vi "ProyectoFinal.vi"() -> ()   [LabVIEW 2020]
uses:
  <vilib>/Instr/_visa.llb/VISA Configure Serial Port (Instr).vi
panel:
  in  "Temperatura Base":string
  out "Unidades de calor":dbl
  in  "Escribir":bool
  in  "Leer":bool
  out "Concentracion de CO":dbl
  out "Temperatura actual":dbl
  out "Humedad actual":dbl
  in  "Temperatura deseada":string
  in  "humedad deseada":string
  in  "VISA resource name":refnum<visa-resource-name>
  in  "stop":bool
  # "INSTITUTO POLITECNICO NACIONAL \nUNIDAD PROFECIONAL INTERDICIPLINARIA DE INGIENERIA CAMPUS ZACATECAS \nPROYECTO: INVERNADERO \nINSTRUMENTACION VIRTUAL"
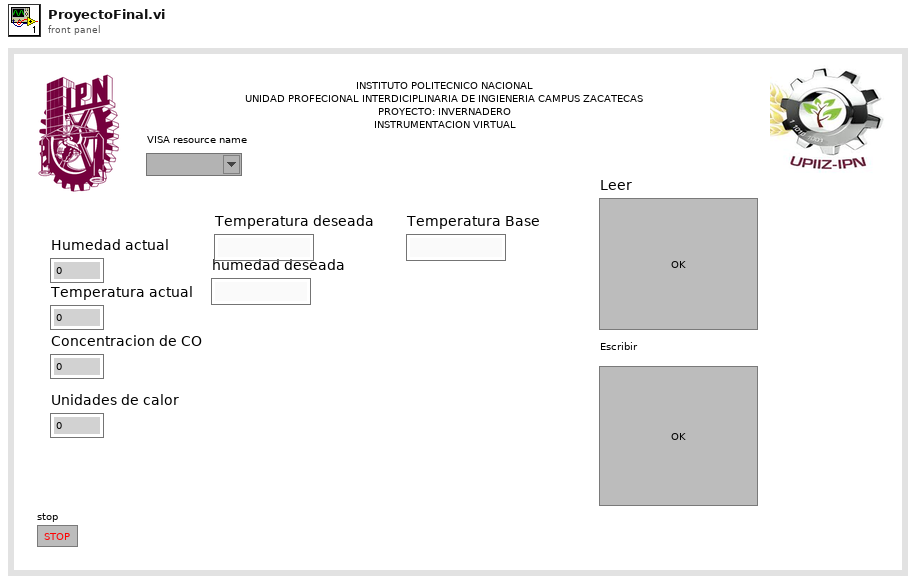
[diagram p1: front panel]
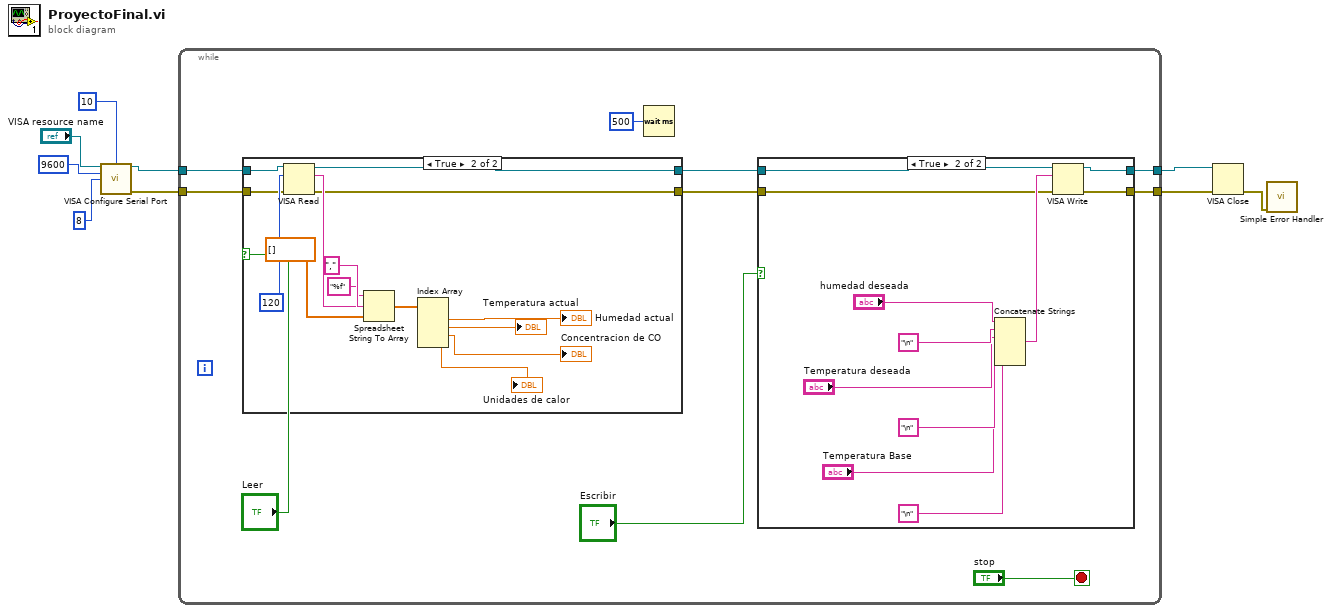
[diagram p0: block diagram]
diagram:
  n1 = call-poly "VISA Configure Serial Port"("VISA resource name"="VISA resource name", "termination char\n(0xA = '\\n' = LF)"=u8 10 ("termination char\n(0xA = '\\n' = LF)"), "baud rate (9600)"=u32 9600, "data bits (8)"=u16 8) -> ("VISA resource name out"=w5:refnum<visa-resource-name>, "error out"=w3:errorcluster)  [unwired: 10 in]
  n2 = while {
    tunnel: w5 -> [w15]
    tunnel: [w13] -> w4
    tunnel: w3 -> [w12]
    tunnel: [w10] -> w2
    stop <- "stop" stop-if-true
    n3 = case shown="True" "Leer" {
      tunnel: w15 -> [w21 w25]
      tunnel: [w21 w24] -> w14
      tunnel: w12 -> [w20 w23]
      tunnel: [w20 w22] -> w11
      frame False {
      }
      frame True {
        n4 = VISA Read(VISA resource name=w25, byte count=u32 120, error in (no error)=w23) -> (VISA resource name out=w24:refnum<visa-resource-name>, read buffer=w29:string, error out=w22:errorcluster)  [unwired: 1 out]
        n5 = Spreadsheet String To Array(delimiter (Tab)=",", format string="%f", spreadsheet string=w29, array type (2D Dbl)=dbl[] []) -> (array=w32:dbl[])
        n6 = Index Array(array=w32) -> (element #1=→"Humedad actual":dbl, element #2=→"Temperatura actual":dbl, element #3=→"Concentracion de CO":dbl, element #4=→"Unidades de calor":dbl)  [unwired: 4 in]
      }
    }
    n7 = Wait (ms)(milliseconds to wait=u32 500) -> ()  [unwired: 1 out]
    n8 = case shown="True" "Escribir" {
      tunnel: w14 -> [w37 w41]
      tunnel: [w37 w40] -> w13
      tunnel: w11 -> [w36 w39]
      tunnel: [w36 w38] -> w10
      frame False {
      }
      frame True {
        n9 = Concatenate Strings("humedad deseada", "\n" ("string"), "Temperatura deseada", "\n" ("string"), "Temperatura Base", "\n" ("string")) -> (w48:string)
        n10 = VISA Write(VISA resource name=w41, write buffer=w48, error in (no error)=w39) -> (VISA resource name out=w40:refnum<visa-resource-name>, error out=w38:errorcluster)  [unwired: 1 out]
      }
    }
  }
  n11 = VISA Close(VISA resource name=w4, error in (no error)=w2) -> (error out=w1:errorcluster)
  n12 = call <vilib>:"Simple Error Handler.vi"("error in (no error)"=w1) -> ()  [unwired: 4 in, 5 out]
